vi "Put Object from file (Multipart).vi"(6 "Chunk size (kB)":i32=5120 min=5120, 7 "Request Parameters":T2={"Content Type"="binary/octet-stream", "ACL"=enum."private", "Storage Class"=enum."STANDARD", "User Metadata"=[]}, 8 "error in (no error)":errorcluster, 9 "Bucket":string, 10 "Object path":string, 11 "Local file path":path) -> (0 "error out":errorcluster, 2 "Version ID":string, 3 "CompleteMultipartUploadResult":T1)   [LabVIEW 2011, in "LV Interface for Amazon S3.lvlib"]
doc: "This operation <B>uploads an object from a file</B> to a bucket <B>in multiple parts</B>. You can <B>set Chunk size (kB) to limit memory usage</B> of the operation."
uses:
  LV Interface for Amazon S3.lvlib
  Typedefs/AMZ_S3_API_POST Multipart Object Request Parameters.ctl
  Typedefs/AMZ_S3_ACL.ctl
  Typedefs/AMZ_S3_Storage Class.ctl
  Typedefs/AMZ_S3_Object Metadata.ctl
  Typedefs/AMZ_S3_API_CompleteMultipartUploadResult.ctl
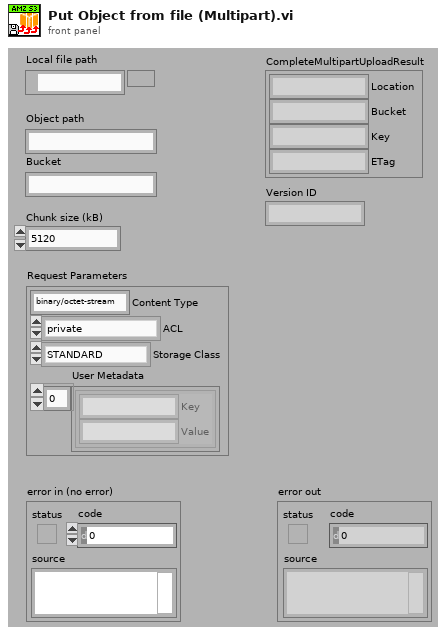
[diagram p1: front panel]
types:
  T1 = typedef "LV Interface for Amazon S3.lvlib/AMZ_S3_API_CompleteMultipartUploadResult.ctl" = cluster{"Location":string, "Bucket":string, "Key":string, "ETag":string}
  T2 = typedef "LV Interface for Amazon S3.lvlib/AMZ_S3_API_POST Multipart Object Request Parameters.ctl" = cluster{"Content Type":string, "ACL":T3, "Storage Class":T4, "User Metadata":T5[]}
  T3 = typedef "LV Interface for Amazon S3.lvlib/AMZ_S3_ACL.ctl" = enum16{"private", "public-read", "public-read-write", "authenticated-read", "bucket-owner-read", "bucket-owner-full-control"}
  T4 = typedef "LV Interface for Amazon S3.lvlib/AMZ_S3_Storage Class.ctl" = enum16{"STANDARD", "REDUCED_REDUNDANCY"}
  T5 = typedef "LV Interface for Amazon S3.lvlib/AMZ_S3_Object Metadata.ctl" = cluster{"Key":string, "Value":string}
  T6 = typedef "LV Interface for Amazon S3.lvlib/AMZ_S3_Multipart Upload RefNum.ctl" = refnum<k1>
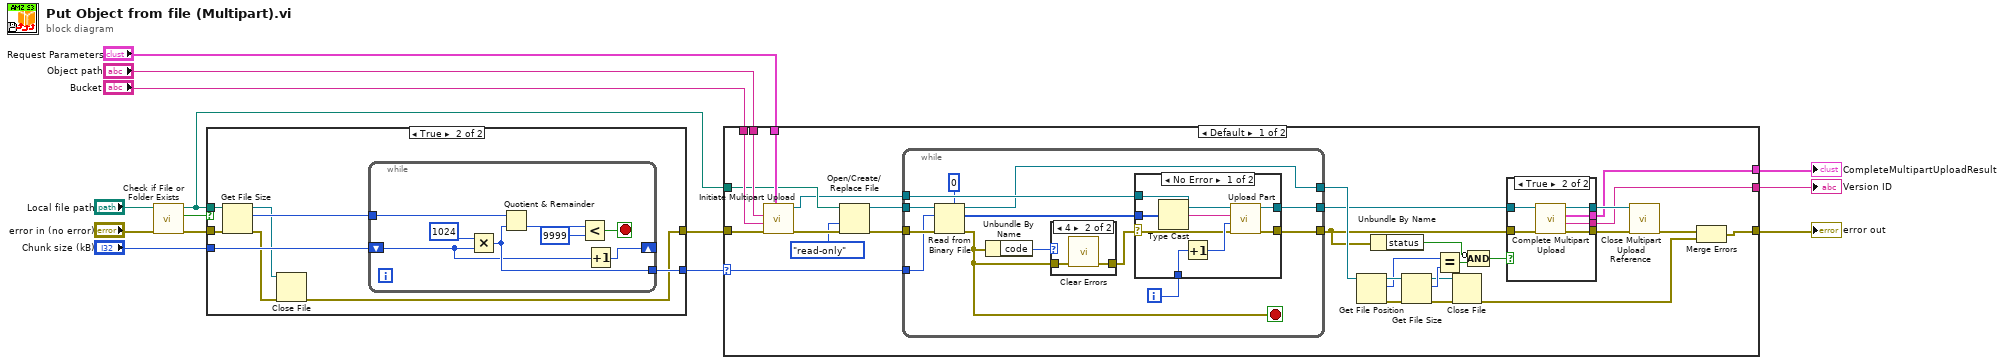
[diagram p0: block diagram]
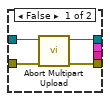
[diagram p2: hidden frame]
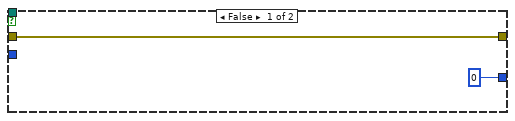
[diagram p6: hidden frame]
diagram:
  n1 = call <vilib>:"Check if File or Folder Exists.vi"("error in (no error)"="error in (no error)", "path"="Local file path") -> ("error out"=w11:errorcluster, "file or folder exists?"=w12:bool, "dup path"=w4:path)  [unwired: 7 in]
  n2 = case shown="True" w12 {
    tunnel: w11 -> [w15 w23]
    tunnel: w4 -> [_ w24]
    tunnel: "Chunk size (kB)" -> [_ w22]
    tunnel: [0 w20] -> w9
    tunnel: [w15 w18] -> w8
    frame False {
    }
    frame True {
      n3 = Get File Size(file=w24, error in=w23) -> (refnum out=w17:refnum<file>, size (in bytes)=w21:i64, 0:w19:errorcluster)
      n4 = Close File(refnum=w17, error in=w19) -> (error out=w18:errorcluster)  [unwired: 1 out]
      n5 = while {
        tunnel: w21 -> [w32]
        shift-right: [w26] -> _
        shift-left: w22 -> [w25]
        tunnel: [w27] -> w20
        stop <- w29 stop-if-true
        n6 = Multiply(x=1024 ("y"), y=w25) -> (x*y=w27:i32)
        n7 = Quotient & Remainder(x=w32, y=w27) -> (floor(x/y)=w31:i64)  [unwired: 1 out]
        n8 = Less?(x=w31, y=i64 9999) -> (x < y?=w29:bool)
        n9 = Increment(x=w25) -> (x+1=w26:i32)
      }
    }
  }
  n10 = case shown="Default" w9 {
    selector: w9 -> [w33 _]
    tunnel: w8 -> [w59 w99]
    tunnel: "Bucket" -> [w62 _]
    tunnel: "Object path" -> [w61 _]
    tunnel: "Request Parameters" -> [w60 _]
    tunnel: w4 -> [w57 _]
    tunnel: [w35 w99] -> w2
    tunnel: [w38 _] -> w3
    tunnel: [w34 _] -> w1
    frame Default {
      n11 = call "Initiate Multipart Upload.vi"("Request Parameters"=w60, "error in (no error)"=w59, "Bucket"=w62, "Path"=w61) -> ("error out"=w58:errorcluster, "Multipart Upload RefNum"=w56:T6)  [unwired: 6 in]
      n12 = Open/Create/Replace File(file path (use dialog)=w57, error in=w58, access (0:read/write)=enum16{"read/write", "read-only", "write-only"}."read-only") -> (refnum out=w53:refnum<file>, error out=w54:errorcluster)  [unwired: 3 in, 1 out]
      n13 = while {
        tunnel: w54 -> [w85]
        tunnel: w53 -> [w84]
        tunnel: w56 -> [w83]
        tunnel: [w74] -> w41
        tunnel: [w73] -> w48
        tunnel: [w82] -> w43
        tunnel: w33 -> [w78]
        i -> [w81]
        stop <- w75 stop-if-true
        n14 = Read from Binary File(5:u8 0, 8:w85, 10:w78, 11:w84) -> (0:w75:errorcluster, 2:w79:u8[], 3:w73:refnum<file>)  [unwired: 2 in, 1 out]
        n15 = Unbundle By Name(w75) -> ("code"=w77:i32)
        n16 = case shown="4" w77 {
          tunnel: w75 -> [w96 w98]
          tunnel: [w96 w97] -> w76
          frame Default {
          }
          frame 4 {
            n17 = call <vilib>:"Clear Errors.vi"("error in (no error)"=w98) -> ("error out"=w97:errorcluster)  [unwired: 6 in]
          }
        }
        n18 = case shown="No Error" w76 {
          selector: w76 -> [w87 w95]
          tunnel: w83 -> [w93 w94]
          tunnel: [w92 w94] -> w82
          tunnel: w81 -> [w91 _]
          tunnel: w79 -> [w89 _]
          tunnel: [w86 w95] -> w74
          frame No Error {
            n19 = Type Cast(x=w89) -> (*(type *) &x=w88:string)  [unwired: 1 in]
            n20 = Increment(x=w91) -> (x+1=w90:i32)
            n21 = call "Upload Part.vi"("error in (no error)"=w87, "Part Number"=w90, "Data"=w88, "Multipart Upload RefNum in"=w93) -> ("error out"=w86:errorcluster, "Multipart Upload RefNum out"=w92:T6)  [unwired: 5 in, 1 out]
          }
          frame Error {
          }
        }
      }
      n22 = Get File Position(7:w48) -> (0:w51:errorcluster, 2:w49:i64, 3:w52:refnum<file>)  [unwired: 1 in]
      n23 = Unbundle By Name(w41) -> ("status"=w45:bool)
      n24 = Get File Size(file=w52, error in=w51) -> (refnum out=w46:refnum<file>, size (in bytes)=w50:i64, 0:w47:errorcluster)
      n25 = Equal?(x=w49, y=w50) -> (x = y?=w44:bool)
      n26 = Close File(refnum=w46, error in=w47) -> (error out=w36:errorcluster)  [unwired: 1 out]
      n27 = Compound Arithmetic op=AND(invert w45, w44) -> (w42:bool)
      n28 = case shown="True" w42 {
        tunnel: w43 -> [w65 w71]
        tunnel: w41 -> [w66 w72]
        tunnel: [w63 w70] -> w40
        tunnel: [_ w69] -> w38
        tunnel: [w64 w68] -> w39
        tunnel: [_ w67] -> w34
        frame False {
          n29 = call "Abort Multipart Upload.vi"("error in (no error)"=w66, "Multipart Upload RefNum in"=w65) -> ("error out"=w63:errorcluster, "Multipart Upload RefNum out"=w64:T6)  [unwired: 7 in, 1 out]
        }
        frame True {
          n30 = call "Complete Multipart Upload.vi"("error in (no error)"=w72, "Multipart Upload RefNum in"=w71) -> ("error out"=w70:errorcluster, "Version ID"=w67:string, "CompleteMultipartUploadResult"=w69:T1, "Multipart Upload RefNum out"=w68:T6)  [unwired: 6 in]
        }
      }
      n31 = call "Close Multipart Upload Reference.vi"("error in (no error)"=w40, "Multipart Upload RefNum in"=w39) -> ("error out"=w37:errorcluster)  [unwired: 9 in]
      n32 = Merge Errors(w37, w36) -> (w35:errorcluster)
    }
    frame 0 {
    }
  }
  "error out" <- w2
  "CompleteMultipartUploadResult" <- w3
  "Version ID" <- w1
